vi "SCCSup Dialog_GenMCLB_SizeColumns.vi"(6 "column index":i32, 8 "error in (no error)":errorcluster, 10 "VI Refnum":refnum<vi>, 11 "Multicolumn Listbox":refnum<vi>) -> (0 "error out":errorcluster, 2 "calc total column width":u32)   [LabVIEW 2020]
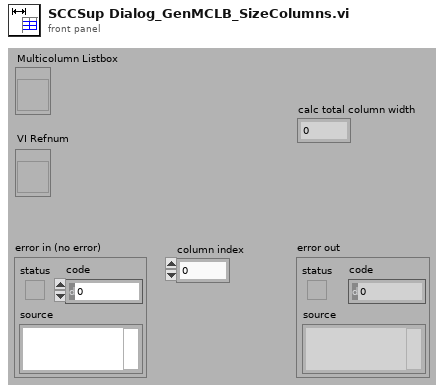
[diagram p1: front panel]
types:
  T1 = enum16{"User-specified Font", "Application Font", "System Font", "Dialog Font"}
  T2 = cluster{"left":i16, "top":i16, "right":i16, "bottom":i16}
  T3 = typedef "LVRowAndColumnUnsignedTypeDef.ctl" = cluster{"Row":u32, "Column":u32}
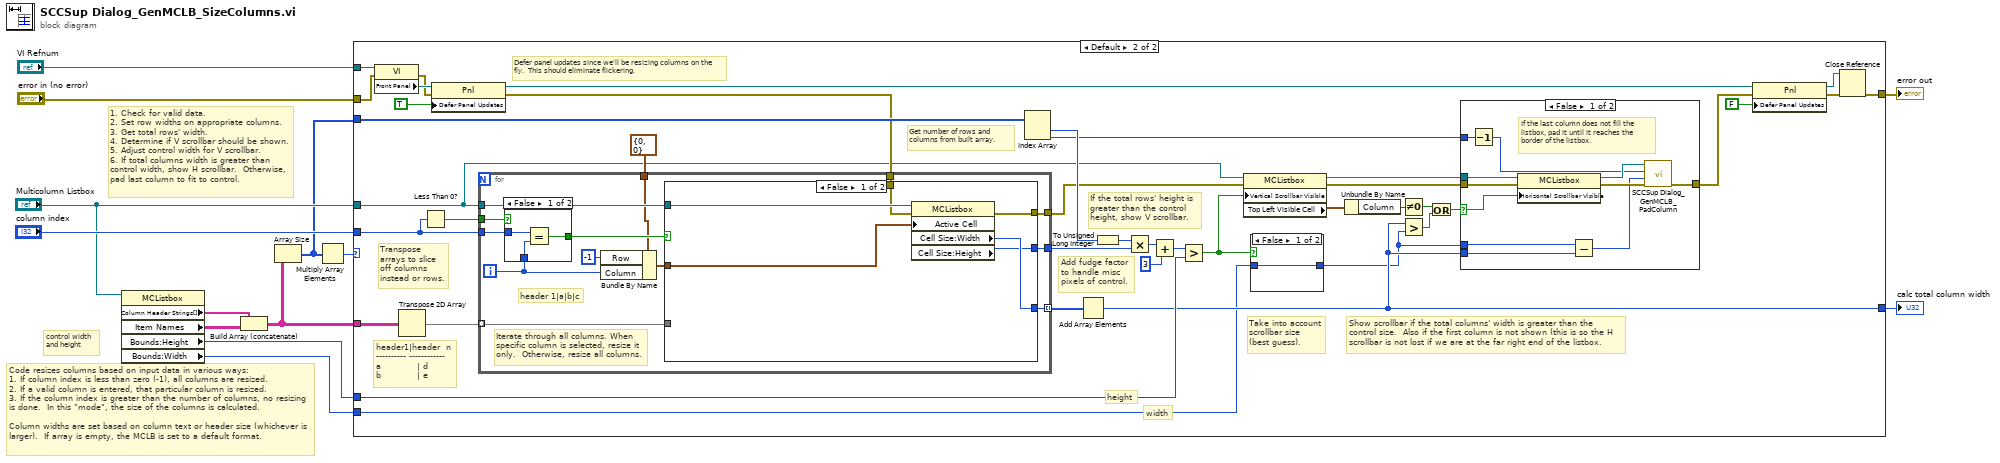
[diagram p0: block diagram]
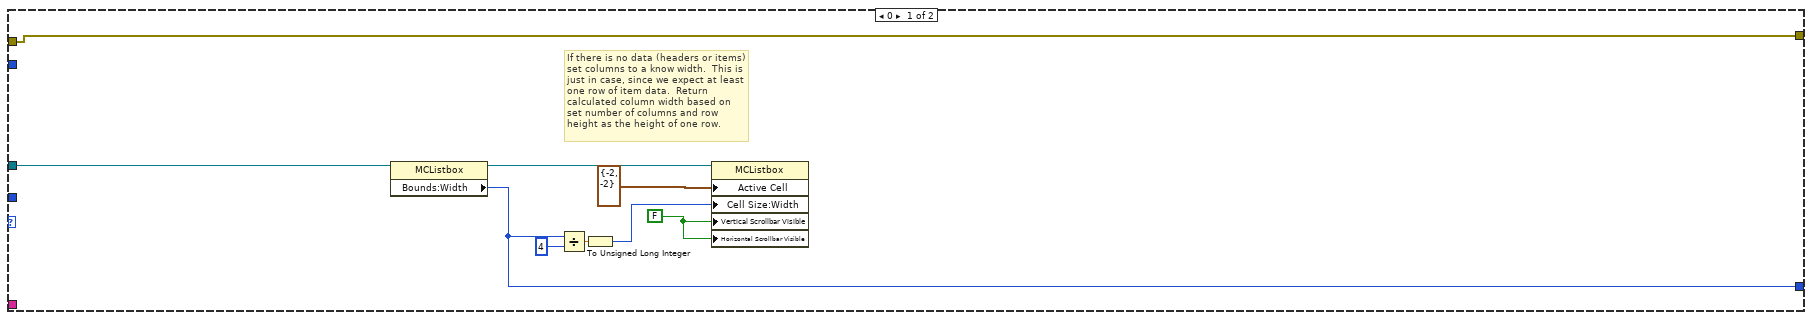
[diagram p2: hidden frame]
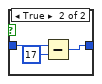
[diagram p3: hidden frame]
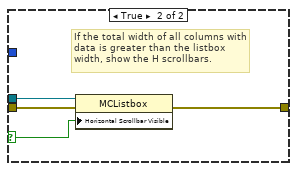
[diagram p4: hidden frame]
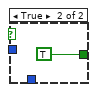
[diagram p5: hidden frame]
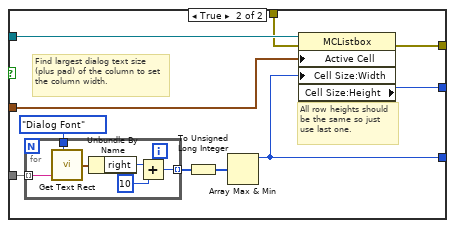
[diagram p6: hidden frame]
diagram:
  # "1. Check for valid data.\n2. Set row widths on appropriate columns.\n3. Get total rows' width.\n4. Determine if V scrollbar should be shown.\n5. Adjust control width for V scrollbar.\n6. If total columns width is greater than control width, show H scrollbar.  Otherwise, pad last column to fit to control."
  # "control width and height"
  # "Code resizes columns based on input data in various ways:\n1. If column index is less than zero (-1), all columns are resized.\n2. If a valid column is entered, that particular column is resized.\n3. If the column index is greater than the number of columns, no resizing is done.  In this \"mode\", the size of the columns is calculated.\n\nColumn widths are set based on column text or header size (whichever is larger).  If array is empty, the MCLB is set to a default format."
  n1 = property on="Property Node" class="MCListbox"(reference="Multicolumn Listbox") -> ("Column Header Strings[]"=w8:string[], "Item Names"=w10:string[][], "Bounds:Height"=w6:u32, "Bounds:Width"=w1:u32)  [unwired: 1 in, 2 out]
  n2 = Build Array (concatenate)(w8, w10) -> (w9:string[][])
  n3 = Array Size(array=w9) -> (size(s)=w5:i32[])
  n4 = Multiply Array Elements(1:w5) -> (0:w7:i32)
  n5 = case shown="Default" w7 {
    tunnel: [w18 w30] -> w12
    tunnel: w9 -> [_ w61]
    tunnel: "Multicolumn Listbox" -> [w20 w34]
    tunnel: "column index" -> [_ w60]
    tunnel: w6 -> [_ w37]
    tunnel: w5 -> [_ w53]
    tunnel: "VI Refnum" -> [_ w48]
    tunnel: "error in (no error)" -> [w21 w46]
    tunnel: [w21 w39] -> w2
    tunnel: w1 -> [_ w29]
    frame 0 {
      w14 = FALSE ("Vertical Scrollbar Visible")
      # "If there is no data (headers or items) set columns to a know width.  This is just in case, since we expect at least one row of item data.  Return calculated column width based on set number of columns and row height as the height of one row."
      n6 = property on="Property Node" class="MCListbox"(reference=w20) -> (reference out=w19:refnum<vi>, "Bounds:Width"=w18:u32)  [unwired: 1 in, 1 out]
      n7 = Divide(x=w18, y=u32 4) -> (x/y=w16:dbl)
      n8 = To Unsigned Long Integer(number=w16) -> (unsigned 32bit integer=w15:u32)
      n9 = property on="Property Node" class="MCListbox"(reference=w19, "Active Cell"=cluster{"Row":i32, "Column":i32} {"Row"=-2, "Column"=-2}, "Cell Size:Width"=w15, "Vertical Scrollbar Visible"=w14, "Horizontal Scrollbar Visible"=w14) -> ()  [unwired: 1 in, 2 out]
    }
    frame Default {
      # "Show scrollbar if the total columns' width is greater than the control size.  Also if the first column is not shown (this is so the H scrollbar is not lost if we are at the far right end of the listbox."
      # "Take into account scrollbar size (best guess)."
      # "width"
      # "height"
      # "If the total rows' height is greater than the control height, show V scrollbar."
      # "Defer panel updates since we'll be resizing columns on the fly.  This should eliminate flickering."
      # "Get number of rows and columns from built array."
      # "header1|header  n\n---------- ------------\na            | d\nb            | e"
      # "Transpose arrays to slice off columns instead or rows."
      # "Add fudge factor to handle misc pixels of control."
      n10 = property class="VI"(reference=w48, error in=w46) -> (error out=w45:errorcluster, "Front Panel"=w50:refnum<vi>)  [unwired: 1 out]
      n11 = Transpose 2D Array(2D array=w61) -> (transposed array=w55:string[][])
      n12 = Less Than 0?(x=w60) -> (x < 0?=w59:bool)
      n13 = property class="Pnl"(reference=w50, error in=w45, "Defer Panel Updates"=TRUE) -> (reference out=w41:refnum<vi>, error out=w47:errorcluster)
      n14 = for {
        tunnel: w55 -> [w92] mode=indexing
        tunnel: [w94] -> w62 mode=indexing
        tunnel: w34 -> [w93]
        tunnel: w60 -> [w90]
        tunnel: w59 -> [w91]
        tunnel: [w85] -> w54
        tunnel: cluster{"Row":i32, "Column":i32} {"Row"=0, "Column"=0} ("Active Cell") -> [w84]
        tunnel: w47 -> [w83]
        tunnel: [w82] -> w36
        i -> [w86]
        # "Iterate through all columns. When specific column is selected, resize it only.  Otherwise, resize all columns."
        # "header 1|a|b|c"
        n15 = case shown="False" w91 {
          tunnel: w90 -> [w96 _]
          tunnel: [w97 TRUE] -> w89
          tunnel: w86 -> [w95 _]
          frame False {
            n16 = Equal?(x=w96, y=w95) -> (x = y?=w97:bool)
          }
          frame True {
          }
        }
        n17 = Bundle By Name(cluster=w84, "Row"=-1, "Column"=w86) -> (w87:cluster{"Row":i32, "Column":i32})
        n18 = case shown="False" w89 {
          tunnel: [w103 w113] -> w94
          tunnel: w93 -> [w104 w112]
          tunnel: w92 -> [_ w110]
          tunnel: w87 -> [w102 w109]
          tunnel: [w101 w108] -> w85
          tunnel: w83 -> [w100 w107]
          tunnel: [w99 w106] -> w82
          frame False {
            n19 = property on="Property Node" class="MCListbox"(reference=w104, error in=w100, "Active Cell"=w102) -> (error out=w99:errorcluster, "Cell Size:Width"=w103:u32, "Cell Size:Height"=w101:u32)  [unwired: 1 out]
          }
          frame True {
            # "All row heights should be the same so just use last one."
            # "Find largest dialog text size (plus pad) of the column to set the column width."
            n20 = for {
              tunnel: w110 -> [w120] mode=indexing
              tunnel: [w116] -> w114 mode=indexing
              tunnel: T1."Dialog Font" ("desired font(Application)") -> [w115]
              n21 = call <vilib>:"Get Text Rect.vi"("desired font(Application)"=w115, "text"=w120) -> ("rect"=w119:T2)  [unwired: 7 in]
              n22 = Unbundle By Name(w119) -> ("right"=w118:i16)
              n23 = Add(x=w118, y=i16 10) -> (x+y=w116:i16)
            }
            n24 = To Unsigned Long Integer(number=w114) -> (unsigned 32bit integer=w111:u32[])
            n25 = Array Max & Min(array=w111) -> (max value=w113:u32)  [unwired: 3 out]
            n26 = property on="Property Node" class="MCListbox"(reference=w112, error in=w107, "Active Cell"=w109, "Cell Size:Width"=w113) -> (error out=w106:errorcluster, "Cell Size:Height"=w108:u32)  [unwired: 1 out]
          }
        }
      }
      n27 = Index Array(array=w53) -> (element #1=w52:i32, element #2=w31:i32)  [unwired: 2 in]
      n28 = Add Array Elements(numeric array=w62) -> (sum=w30:u32)
      n29 = To Unsigned Long Integer(number=w52) -> (unsigned 32bit integer=w56:u32)
      n30 = Multiply(x=w56, y=w54) -> (x*y=w57:u32)
      n31 = Add(x=w57, y=u32 3 ("x")) -> (x+y=w38:u32)
      n32 = Greater?(x=w38, y=w37) -> (0:w32:bool)
      n33 = property on="Property Node" class="MCListbox"(reference=w34, error in=w36, "Vertical Scrollbar Visible"=w32) -> (reference out=w33:refnum<vi>, error out=w35:errorcluster, "Top Left Visible Cell"=w27:T3)
      n34 = case shown="False" w32 {
        tunnel: w29 -> [w63 w66]
        tunnel: [w63 w64] -> w28
        frame False {
        }
        frame True {
          n35 = Subtract(x=w66, y=u32 17) -> (x-y=w64:u32)
        }
      }
      n36 = Unbundle By Name(w27) -> ("Column"=w26:u32)
      n37 = Not Equal To 0?(x=w26) -> (x != 0?=w24:bool)
      n38 = Greater?(x=w30, y=w28) -> (0:w25:bool)
      n39 = Or(x=w24, y=w25) -> (x .or. y?=w23:bool)
      n40 = case shown="False" w23 {
        selector: w23 -> [w72 w78]
        tunnel: w31 -> [w77 _]
        tunnel: w33 -> [w75 w80]
        tunnel: w35 -> [w74 w81]
        tunnel: [w76 w79] -> w40
        tunnel: w30 -> [w68 _]
        tunnel: w28 -> [w67 _]
        frame False {
          # "If the last column does not fill the listbox, pad it until it reaches the border of the listbox."
          n41 = Decrement(x=w77) -> (x-1=w70:i32)
          n42 = property on="Property Node" class="MCListbox"(reference=w75, error in=w74, "Horizontal Scrollbar Visible"=w72) -> (reference out=w71:refnum<vi>, error out=w73:errorcluster)
          n43 = Subtract(x=w67, y=w68) -> (x-y=w69:u32)
          n44 = call <vilib>:"SCCSup Dialog_GenMCLB_PadColumn.vi"("error in (no error)"=w73, "padding"=w69, "column"=w70, "multicolumn listbox"=w71) -> ("error out"=w76:errorcluster)  [unwired: 7 in]
        }
        frame True {
          # "If the total width of all columns with data is greater than the listbox width, show the H scrollbars."
          n45 = property on="Property Node" class="MCListbox"(reference=w80, error in=w81, "Horizontal Scrollbar Visible"=w78) -> (error out=w79:errorcluster)  [unwired: 1 out]
        }
      }
      n46 = property class="Pnl"(reference=w41, error in=w40, "Defer Panel Updates"=FALSE) -> (reference out=w44:refnum<vi>, error out=w43:errorcluster)
      n47 = Close Reference(reference=w44, error in (no error)=w43) -> (error out=w39:errorcluster)
    }
  }
  "calc total column width" <- w12
  "error out" <- w2
